vi "Begin.vi"() -> (0 "error out":errorcluster)   [LabVIEW 2014]
doc: "Called before other user functions, this VI is expected to open initial I/O refnums, load in file data, and do all program initialization. Notice that the <B>error out</B> terminal is simply used for data flow. Wiring it to other structures or subVIs ensures that this VI runs first."
uses:
  <vilib>/Rock Robotics/WPI/DriverStation/WPI_DriverStationRobotMode2.ctl
  <vilib>/Rock Robotics/WPI/Joystick/WPI_JoystickDeviceEnum.ctl
  <vilib>/Rock Robotics/SystemInterfaces/DIO/FPGA_DIOPWMChannel.ctl
  <vilib>/Rock Robotics/SystemInterfaces/DIO/FPGA_DIOChannel.ctl
  <vilib>/Rock Robotics/WPI/Solenoid/WPI_SolenoidChannel.ctl
  <vilib>/Rock Robotics/SystemInterfaces/AI/FPGA_AIGyroChannel.ctl
  Robot Global Data.vi
  <vilib>/Rock Robotics/Network Tables/SD Write String Array.vi
  <vilib>/Rock Robotics/WPI/MotorControl/WPI_MotorControlOpen Talon.vi
  <vilib>/Rock Robotics/WPI/Counter/WPI_CounterDigitalInputToDigitalSource.vi
  <vilib>/Rock Robotics/WPI/Solenoid/WPI_SolenoidOpenDouble.vi
  Global Variables/Refnum Names.vi
  Global Variables/Calibrations.vi
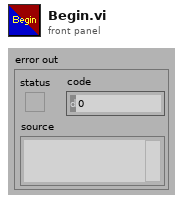
[diagram p1: front panel]
types:
  T1 = typedef "FPGA_DIOChannel.ctl" = enum8{"DIO 0", "DIO 1", "DIO 2", "DIO 3", "DIO 4", "DIO 5", "DIO 6", "DIO 7", "DIO 8", "DIO 9", "DIO MXP 0", "DIO MXP 1", "DIO MXP 2", "DIO MXP 3", "DIO MXP 4", "DIO MXP 5", "DIO MXP 6", "DIO MXP 7", "DIO MXP 8", "DIO MXP 9", "DIO MXP 10", "DIO MXP 11", "DIO MXP 12", "DIO MXP 13", "DIO MXP 14", "DIO MXP 15", "Invalid"}
  T2 = typedef "FPGA_DIOPWMChannel.ctl" = enum8{"PWM 0", "PWM 1", "PWM 2", "PWM 3", "PWM 4", "PWM 5", "PWM 6", "PWM 7", "PWM 8", "PWM 9", "PWM MXP 0", "PWM MXP 1", "PWM MXP 2", "PWM MXP 3", "PWM MXP 4", "PWM MXP 5", "PWM MXP 6", "PWM MXP 7", "PWM MXP 8", "PWM MXP 9", "Invalid"}
  T3 = typedef "WPI_JoystickDeviceEnum.ctl" = enum16{"USB 0", "USB 1", "USB 2", "USB 3", "USB 4", "USB 5"}
  T4 = typedef "FPGA_AIGyroChannel.ctl" = enum8{"AI 0", "AI 1", "Invalid"}
  T5 = typedef "WPI_SolenoidChannel.ctl" = enum8{"Solenoid 0", "Solenoid 1", "Solenoid 2", "Solenoid 3", "Solenoid 4", "Solenoid 5", "Solenoid 6", "Solenoid 7", "Invalid"}
  T6 = typedef "WPI_DriverStationRobotMode2.ctl" = enum16{"Autonomous Disabled", "Autonomous Enabled", "Teleop Disabled", "Teleop Enabled", "Disconnected", "Finish", "Test Disabled", "Test Enabled", "Emergency Stopped"}
  T7 = typedef "WPI_MotorControlDeviceRef.ctl" = cluster{"DeviceStatus":errorcluster, "Type":T8, "PWM":cluster{"Controller":T9, "PWM Channel":T2, "DeadBand":T10}, "CAN":cluster{"Device Number":u8, "Control Mode":T11, "Semaphore":T12, "Max Vout":dbl, "TalonSRX Control Mode":T13}, "Invert":bool, "TransformRef":T14, "InvTransformRef":T14}
  T8 = typedef "WPI_MotorControlType.ctl" = enum16{"PWM", "CAN", "CANTalonSRX"}
  T9 = typedef "FPGA_TypedefDigitalModule.ctl" = enum16{"Controller 1"}
  T10 = typedef "WPI_PWMDeadband.ctl" = cluster{"Name":string, "maxPositivePwm":i32, "minPositivePwm":i32, "centerPwm":i32, "maxNegativePwm":i32, "minNegativePwm":i32, "angularRange":u16}
  T11 = typedef "WPI_CANJaguar_ControlMode.ctl" = enum8{"Percent VBus", "Current", "Speed", "Position", "Voltage"}
  T12 = typedef "Semaphore RefNum" = refnum<k1>
  T13 = typedef "WPI_CANTalonSRX_APIControlMode.ctl" = enum8{"Percent VBus", "Speed", "Position", "Slave", "Unchanged / Invalid"}
  T14 = typedef "WPI_PWMTransform_ConPane.ctl" = refnum<vi>
  T15 = typedef "WPI_ServoDeviceRef.ctl" = cluster{"DeviceStatus":errorcluster, "Controller":T9, "PWM Channel":T2, "DeadBand":T10}
  T16 = typedef "WPI_JoystickDevRef.ctl" = cluster{"Device":T3}
  T17 = typedef "WPI_DigitalInputDevRef.ctl" = cluster{"DevStatus":errorcluster, "DIO Channel":T1, "Controller":T9}
  T18 = typedef "FPGA_CounterEncoderSourceConvertionLVSourceType.ctl" = cluster{"DevStatus":errorcluster, "AnalogTriggerMode?":bool, "DigitalMode":cluster{"Controller":T9, "DIO Channel":T19}, "AnalogTriggerMode":cluster{"AnalogTriggerIndex":T20, "OutputType":T21}}
  T19 = typedef "FPGA_DIODigitalSourceChannel.ctl" = enum8{"DIO 0", "DIO 1", "DIO 2", "DIO 3", "DIO 4", "DIO 5", "DIO 6", "DIO 7", "DIO 8", "DIO 9", "DIO MXP 0", "DIO MXP 1", "DIO MXP 2", "DIO MXP 3", "DIO MXP 4", "DIO MXP 5", "DIO MXP 6", "DIO MXP 7", "DIO MXP 8", "DIO MXP 9", "DIO MXP 10", "DIO MXP 11", "DIO MXP 12", "DIO MXP 13", "DIO MXP 14", "DIO MXP 15", "Disabled"}
  T20 = typedef "FPGA_AnalogTriggerIndex.ctl" = enum8{"Trig 0", "Trig 1", "Trig 2", "Trig 3", "Trig 4", "Trig 5", "Trig 6", "Trig 7", "Invalid"}
  T21 = typedef "FPGA_AnalogTriggerOutType.ctl" = enum16{"InWindow", "TriggerState", "Rising", "Falling"}
  T22 = typedef "WPI_EncoderDevRef.ctl" = cluster{"DevStatus":errorcluster, "EncoderIndex":T23, "CounterIndex":T24, "DistancePerCount":dbl, "Decoding Type":T25}
  T23 = typedef "FPGA_EncoderIdx.ctl" = enum8{"Enc 0", "Enc 1", "Enc 2", "Enc 3", "Enc 4", "Enc 5", "Enc 6", "Enc 7", "Invalid"}
  T24 = typedef "FPGA_CounterCtrSystemIndex.ctl" = enum8{"Ctr 0", "Ctr 1", "Ctr 2", "Ctr 3", "Ctr 4", "Ctr 5", "Ctr 6", "Ctr 7", "Invalid"}
  T25 = typedef "WPI_EncoderType.ctl" = enum16{"1x", "2x", "4x"}
  T26 = typedef "WPI_SolenoidDevRef.ctl" = cluster{"DevStatus":errorcluster, "Pneumatics Control Module":u8, "Forward Solenoid Channel":T5, "Reverse Solenoid Channel":T5}
  T27 = typedef "WPI_GyroDevRef.ctl" = cluster{"DevStatus":errorcluster, "Analog Module":T28, "Analog Channel":T29, "Offset":dbl, "Gain (VoltsPerDegree/Second)":dbl}
  T28 = typedef "FPGA_TypedefAnalogModule.ctl" = enum16{"Controller 1"}
  T29 = typedef "FPGA_AIChannel.ctl" = enum8{"AI 0", "AI 1", "AI 2", "AI 3", "AI MXP 0", "AI MXP 1", "AI MXP 2", "AI MXP 3", "Invalid"}
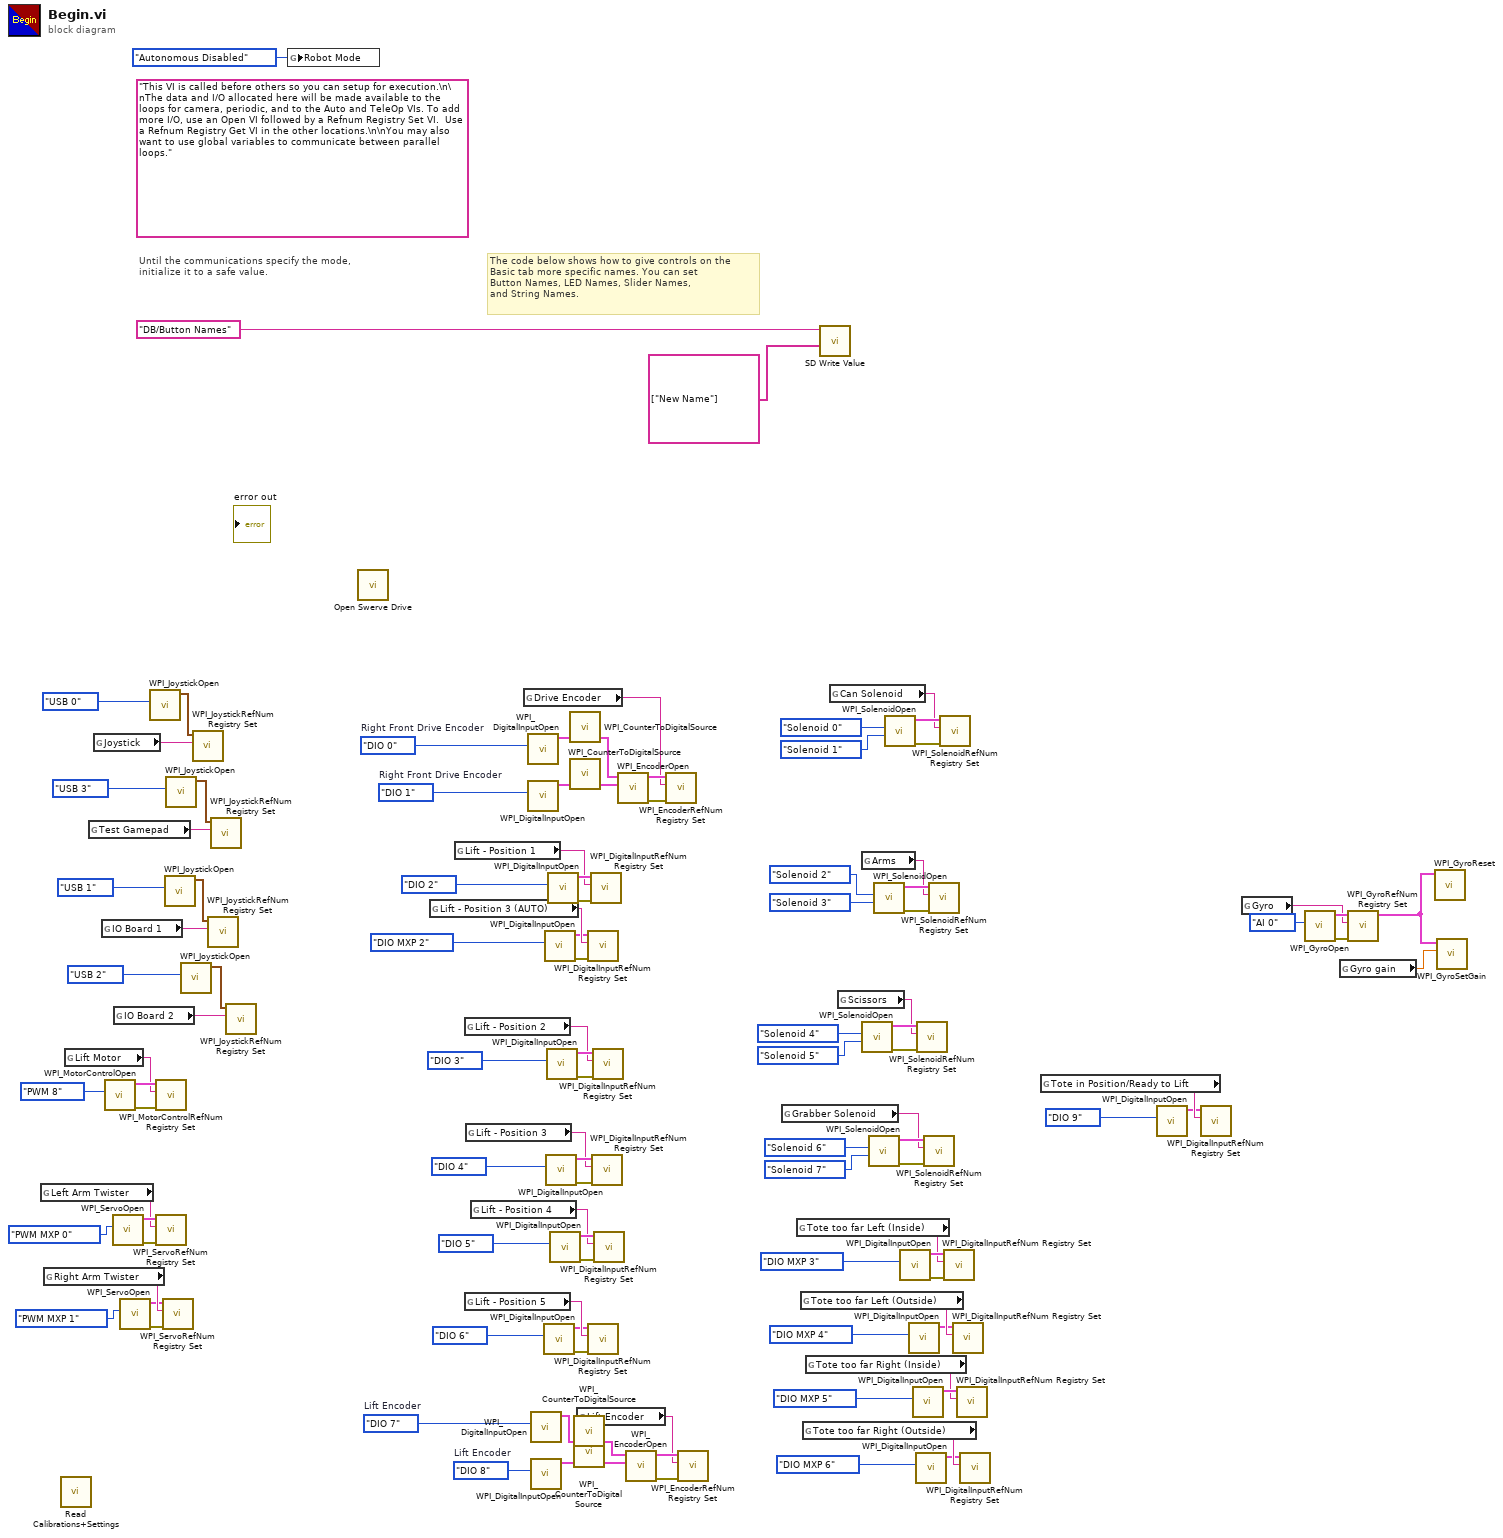
[diagram p0: block diagram]
diagram:
  w75 = FPGA_DIOChannel."DIO 8"  # Lift Encoder
  w74 = FPGA_DIOChannel."DIO 7"  # Lift Encoder
  w96 = FPGA_DIOChannel."DIO 1"  # Right Front Drive Encoder
  w95 = FPGA_DIOChannel."DIO 0"  # Right Front Drive Encoder
  (unwired) "This VI is called before others so you can setup for execution.\n\nThe data and I/O allocated here will be made available to the loops for camera, periodic, and to the Auto and TeleOp VIs. To add more I/O, use an Open VI followed by a Refnum Registry Set VI.  Use a Refnum Registry Get VI in the other locations.\n\nYou may also want to use global variables to communicate between parallel loops."
  # "The code below shows how to give controls on the\nBasic tab more specific names. You can set\nButton Names, LED Names, Slider Names,\nand String Names."
  # "Until the communications specify the mode,\ninitialize it to a safe value."
  n1 = global read "Refnum Names.vi" "Left Arm Twister"() -> (w98:string)
  n2 = global read "Refnum Names.vi" "Right Arm Twister"() -> (w18:string)
  n3 = call "Read Calibrations+Settings.vi"() -> ()  [unwired: 12 in]
  n4 = global read "Refnum Names.vi" "Lift Motor"() -> (w97:string)
  n5 = global read "Refnum Names.vi" "Test Gamepad"() -> (w105:string)
  n6 = global read "Refnum Names.vi" "Joystick"() -> (w103:string)
  n7 = global read "Refnum Names.vi" "IO Board 1"() -> (w26:string)
  n8 = call-poly <vilib>:"WPI_MotorControlOpen.vi"("PWM Channel"=FPGA_DIOPWMChannel."PWM 8") -> ("error out"=w100:errorcluster, "MotorControlDeviceRef"=w101:T7)  [unwired: 9 in]
  n9 = call <vilib>:"WPI_ServoOpen.vi"("PWM Channel"=FPGA_DIOPWMChannel."PWM MXP 0") -> ("error out"=w42:errorcluster, "ServoDeviceRef"=w99:T15)  [unwired: 9 in]
  n10 = global read "Refnum Names.vi" "IO Board 2"() -> (w24:string)
  n11 = call <vilib>:"WPI_ServoOpen.vi"("PWM Channel"=FPGA_DIOPWMChannel."PWM MXP 1") -> ("error out"=w20:errorcluster, "ServoDeviceRef"=w17:T15)  [unwired: 9 in]
  n12 = call <vilib>:"WPI_JoystickOpen.vi"("JoystickDevice"=WPI_JoystickDeviceEnum."USB 0") -> ("JoystickDevRef"=w104:T16)  [unwired: 10 in]
  n13 = call <vilib>:"WPI_MotorControlRefNum Registry Set.vi"("error in (no error)"=w100, "refnum name"=w97, "MotorControlDevRef"=w101) -> ()  [unwired: 7 in, 2 out]
  n14 = call <vilib>:"WPI_ServoRefNum Registry Set.vi"("error in (no error)"=w42, "refnum name"=w98, "ServoDeviceRef"=w99) -> ()  [unwired: 7 in, 2 out]
  n15 = call <vilib>:"WPI_ServoRefNum Registry Set.vi"("error in (no error)"=w20, "refnum name"=w18, "ServoDeviceRef"=w17) -> ()  [unwired: 7 in, 2 out]
  n16 = call <vilib>:"WPI_JoystickOpen.vi"("JoystickDevice"=WPI_JoystickDeviceEnum."USB 1") -> ("JoystickDevRef"=w25:T16)  [unwired: 10 in]
  n17 = call <vilib>:"WPI_JoystickOpen.vi"("JoystickDevice"=WPI_JoystickDeviceEnum."USB 3") -> ("JoystickDevRef"=w106:T16)  [unwired: 10 in]
  n18 = call <vilib>:"WPI_JoystickOpen.vi"("JoystickDevice"=WPI_JoystickDeviceEnum."USB 2") -> ("JoystickDevRef"=w23:T16)  [unwired: 10 in]
  n19 = call <vilib>:"WPI_JoystickRefNum Registry Set.vi"("refnum name"=w103, "JoystickDevRef"=w104) -> ()  [unwired: 8 in, 2 out]
  n20 = call <vilib>:"WPI_JoystickRefNum Registry Set.vi"("refnum name"=w26, "JoystickDevRef"=w25) -> ()  [unwired: 8 in, 2 out]
  n21 = call <vilib>:"WPI_JoystickRefNum Registry Set.vi"("refnum name"=w105, "JoystickDevRef"=w106) -> ()  [unwired: 8 in, 2 out]
  n22 = call <vilib>:"WPI_JoystickRefNum Registry Set.vi"("refnum name"=w24, "JoystickDevRef"=w23) -> ()  [unwired: 8 in, 2 out]
  n23 = global write "Robot Global Data.vi" "Robot Mode"(WPI_DriverStationRobotMode2."Autonomous Disabled" ("Robot Mode")) -> ()
  n24 = call "Open Swerve Drive.vi"() -> ()  [unwired: 12 in]
  n25 = global read "Refnum Names.vi" "Lift - Position 3 (AUTO)"() -> (w16:string)
  n26 = global read "Refnum Names.vi" "Lift - Position 1"() -> (w41:string)
  n27 = global read "Refnum Names.vi" "Lift - Position 2"() -> (w40:string)
  n28 = global read "Refnum Names.vi" "Lift - Position 5"() -> (w37:string)
  n29 = global read "Refnum Names.vi" "Lift - Position 3"() -> (w39:string)
  n30 = global read "Refnum Names.vi" "Lift - Position 4"() -> (w38:string)
  n31 = global read "Refnum Names.vi" "Drive Encoder"() -> (w88:string)
  n32 = call <vilib>:"WPI_DigitalInputOpen.vi"("DIO Channel"=w95) -> ("DigitalInputDevRef"=w93:T17)  [unwired: 2 in, 8 out]
  n33 = call <vilib>:"WPI_DigitalInputOpen.vi"("DIO Channel"=w96) -> ("DigitalInputDevRef"=w94:T17)  [unwired: 2 in, 8 out]
  n34 = call <vilib>:"WPI_DigitalInputOpen.vi"("DIO Channel"=w74) -> ("DigitalInputDevRef"=w72:T17)  [unwired: 2 in, 8 out]
  n35 = call <vilib>:"WPI_DigitalInputOpen.vi"("DIO Channel"=w75) -> ("DigitalInputDevRef"=w73:T17)  [unwired: 2 in, 8 out]
  n36 = call <vilib>:"WPI_DigitalInputOpen.vi"("DIO Channel"=FPGA_DIOChannel."DIO 6") -> ("error out"=w35:errorcluster, "DigitalInputDevRef"=w34:T17)  [unwired: 9 in]
  n37 = call <vilib>:"WPI_DigitalInputOpen.vi"("DIO Channel"=FPGA_DIOChannel."DIO MXP 2") -> ("error out"=w14:errorcluster, "DigitalInputDevRef"=w13:T17)  [unwired: 9 in]
  n38 = call <vilib>:"WPI_DigitalInputOpen.vi"("DIO Channel"=FPGA_DIOChannel."DIO 4") -> ("error out"=w80:errorcluster, "DigitalInputDevRef"=w81:T17)  [unwired: 9 in]
  n39 = call <vilib>:"WPI_DigitalInputOpen.vi"("DIO Channel"=FPGA_DIOChannel."DIO 3") -> ("error out"=w83:errorcluster, "DigitalInputDevRef"=w84:T17)  [unwired: 9 in]
  n40 = call <vilib>:"WPI_DigitalInputOpen.vi"("DIO Channel"=FPGA_DIOChannel."DIO 2") -> ("error out"=w86:errorcluster, "DigitalInputDevRef"=w87:T17)  [unwired: 9 in]
  n41 = call <vilib>:"WPI_DigitalInputOpen.vi"("DIO Channel"=FPGA_DIOChannel."DIO 5") -> ("error out"=w77:errorcluster, "DigitalInputDevRef"=w78:T17)  [unwired: 9 in]
  n42 = call-poly <vilib>:"WPI_CounterToDigitalSource.vi"("DigitalInputDevRef"=w93) -> ("Digital Source"=w92:T18)  [unwired: 6 out]
  n43 = call-poly <vilib>:"WPI_CounterToDigitalSource.vi"("DigitalInputDevRef"=w94) -> ("Digital Source"=w91:T18)  [unwired: 6 out]
  n44 = call-poly <vilib>:"WPI_CounterToDigitalSource.vi"("DigitalInputDevRef"=w72) -> ("Digital Source"=w71:T18)  [unwired: 6 out]
  n45 = call-poly <vilib>:"WPI_CounterToDigitalSource.vi"("DigitalInputDevRef"=w73) -> ("Digital Source"=w70:T18)  [unwired: 6 out]
  n46 = global read "Refnum Names.vi" "Lift Encoder"() -> (w67:string)
  n47 = call <vilib>:"WPI_DigitalInputRefNum Registry Set.vi"("error in (no error)"=w14, "refnum name"=w16, "DigitalInputDevRef"=w13) -> ()  [unwired: 7 in, 2 out]
  n48 = call <vilib>:"WPI_DigitalInputRefNum Registry Set.vi"("error in (no error)"=w35, "refnum name"=w37, "DigitalInputDevRef"=w34) -> ()  [unwired: 7 in, 2 out]
  n49 = call <vilib>:"WPI_DigitalInputRefNum Registry Set.vi"("error in (no error)"=w86, "refnum name"=w41, "DigitalInputDevRef"=w87) -> ()  [unwired: 7 in, 2 out]
  n50 = call <vilib>:"WPI_DigitalInputRefNum Registry Set.vi"("error in (no error)"=w80, "refnum name"=w39, "DigitalInputDevRef"=w81) -> ()  [unwired: 7 in, 2 out]
  n51 = call <vilib>:"WPI_DigitalInputRefNum Registry Set.vi"("error in (no error)"=w83, "refnum name"=w40, "DigitalInputDevRef"=w84) -> ()  [unwired: 7 in, 2 out]
  n52 = call <vilib>:"WPI_DigitalInputRefNum Registry Set.vi"("error in (no error)"=w77, "refnum name"=w38, "DigitalInputDevRef"=w78) -> ()  [unwired: 7 in, 2 out]
  n53 = call <vilib>:"WPI_EncoderOpen.vi"("BSource"=w91, "ASource"=w92) -> ("error out"=w89:errorcluster, "EncoderDevRef"=w90:T22)  [unwired: 6 in, 2 out]
  n54 = call <vilib>:"WPI_EncoderOpen.vi"("BSource"=w70, "ASource"=w71) -> ("error out"=w68:errorcluster, "EncoderDevRef"=w69:T22)  [unwired: 6 in, 2 out]
  n55 = call <vilib>:"WPI_EncoderRefNum Registry Set.vi"("error in (no error)"=w89, "refnum name"=w88, "EncoderDevRef"=w90) -> ()  [unwired: 7 in, 2 out]
  n56 = call <vilib>:"WPI_EncoderRefNum Registry Set.vi"("error in (no error)"=w68, "refnum name"=w67, "EncoderDevRef"=w69) -> ()  [unwired: 7 in, 2 out]
  n57 = global read "Refnum Names.vi" "Grabber Solenoid"() -> (w44:string)
  n58 = global read "Refnum Names.vi" "Tote too far Left (Inside)"() -> (w30:string)
  n59 = global read "Refnum Names.vi" "Tote too far Left (Outside)"() -> (w12:string)
  n60 = global read "Refnum Names.vi" "Tote too far Right (Outside)"() -> (w6:string)
  n61 = global read "Refnum Names.vi" "Tote too far Right (Inside)"() -> (w7:string)
  n62 = call-poly <vilib>:"SD Write Value.vi"("String Array"=string[] ["New Name"], "Name"="DB/Button Names") -> ()  [unwired: 8 in, 2 out]
  n63 = global read "Refnum Names.vi" "Can Solenoid"() -> (w59:string)
  n64 = global read "Refnum Names.vi" "Scissors"() -> (w49:string)
  n65 = global read "Refnum Names.vi" "Arms"() -> (w54:string)
  n66 = call-poly <vilib>:"WPI_SolenoidOpen.vi"("Reverse Solenoid Channel"=WPI_SolenoidChannel."Solenoid 5", "Forward Solenoid Channel"=WPI_SolenoidChannel."Solenoid 4" ("Solenoid Channel")) -> ("error out"=w53:errorcluster, "SolenoidDevRef"=w52:T26)  [unwired: 8 in]
  n67 = call-poly <vilib>:"WPI_SolenoidOpen.vi"("Reverse Solenoid Channel"=WPI_SolenoidChannel."Solenoid 7", "Forward Solenoid Channel"=WPI_SolenoidChannel."Solenoid 6" ("Solenoid Channel")) -> ("error out"=w48:errorcluster, "SolenoidDevRef"=w47:T26)  [unwired: 8 in]
  n68 = call-poly <vilib>:"WPI_SolenoidOpen.vi"("Reverse Solenoid Channel"=WPI_SolenoidChannel."Solenoid 3", "Forward Solenoid Channel"=WPI_SolenoidChannel."Solenoid 2" ("Solenoid Channel")) -> ("error out"=w58:errorcluster, "SolenoidDevRef"=w57:T26)  [unwired: 8 in]
  n69 = call-poly <vilib>:"WPI_SolenoidOpen.vi"("Reverse Solenoid Channel"=WPI_SolenoidChannel."Solenoid 1", "Forward Solenoid Channel"=WPI_SolenoidChannel."Solenoid 0" ("Solenoid Channel")) -> ("error out"=w63:errorcluster, "SolenoidDevRef"=w62:T26)  [unwired: 8 in]
  n70 = call <vilib>:"WPI_DigitalInputOpen.vi"("DIO Channel"=FPGA_DIOChannel."DIO MXP 3") -> ("error out"=w32:errorcluster, "DigitalInputDevRef"=w33:T17)  [unwired: 9 in]
  n71 = call <vilib>:"WPI_DigitalInputOpen.vi"("DIO Channel"=FPGA_DIOChannel."DIO MXP 4") -> ("DigitalInputDevRef"=w10:T17)  [unwired: 9 in, 1 out]
  n72 = call <vilib>:"WPI_DigitalInputOpen.vi"("DIO Channel"=FPGA_DIOChannel."DIO MXP 5") -> ("DigitalInputDevRef"=w9:T17)  [unwired: 9 in, 1 out]
  n73 = call <vilib>:"WPI_DigitalInputOpen.vi"("DIO Channel"=FPGA_DIOChannel."DIO MXP 6") -> ("DigitalInputDevRef"=w4:T17)  [unwired: 9 in, 1 out]
  n74 = call <vilib>:"WPI_SolenoidRefNum Registry Set.vi"("error in (no error)"=w53, "refnum name"=w49, "SolenoidDevRef"=w52) -> ()  [unwired: 7 in, 2 out]
  n75 = call <vilib>:"WPI_SolenoidRefNum Registry Set.vi"("error in (no error)"=w48, "refnum name"=w44, "SolenoidDevRef"=w47) -> ()  [unwired: 7 in, 2 out]
  n76 = call <vilib>:"WPI_SolenoidRefNum Registry Set.vi"("error in (no error)"=w58, "refnum name"=w54, "SolenoidDevRef"=w57) -> ()  [unwired: 7 in, 2 out]
  n77 = call <vilib>:"WPI_SolenoidRefNum Registry Set.vi"("error in (no error)"=w63, "refnum name"=w59, "SolenoidDevRef"=w62) -> ()  [unwired: 7 in, 2 out]
  n78 = call <vilib>:"WPI_DigitalInputRefNum Registry Set.vi"("error in (no error)"=w32, "refnum name"=w30, "DigitalInputDevRef"=w33) -> ()  [unwired: 7 in, 2 out]
  n79 = call <vilib>:"WPI_DigitalInputRefNum Registry Set.vi"("refnum name"=w12, "DigitalInputDevRef"=w10) -> ()  [unwired: 8 in, 2 out]
  n80 = call <vilib>:"WPI_DigitalInputRefNum Registry Set.vi"("refnum name"=w7, "DigitalInputDevRef"=w9) -> ()  [unwired: 8 in, 2 out]
  n81 = call <vilib>:"WPI_DigitalInputRefNum Registry Set.vi"("refnum name"=w6, "DigitalInputDevRef"=w4) -> ()  [unwired: 8 in, 2 out]
  n82 = global read "Refnum Names.vi" "Tote in Position/Ready to Lift"() -> (w3:string)
  n83 = call <vilib>:"WPI_DigitalInputOpen.vi"("DIO Channel"=FPGA_DIOChannel."DIO 9") -> ("DigitalInputDevRef"=w1:T17)  [unwired: 9 in, 1 out]
  n84 = call <vilib>:"WPI_DigitalInputRefNum Registry Set.vi"("refnum name"=w3, "DigitalInputDevRef"=w1) -> ()  [unwired: 8 in, 2 out]
  n85 = global read "Refnum Names.vi" "Gyro"() -> (w64:string)
  n86 = call <vilib>:"WPI_GyroOpen.vi"("Analog Channel"=FPGA_AIGyroChannel."AI 0") -> ("error out"=w66:errorcluster, "GyroDevRef"=w65:T27)  [unwired: 8 in, 1 out]
  n87 = global read "Calibrations.vi" "Gyro gain"() -> (w27:dbl)
  n88 = call <vilib>:"WPI_GyroRefNum Registry Set.vi"("error in (no error)"=w66, "refnum name"=w64, "GyroDevRef"=w65) -> ("GyroDevRef"=w28:T27)  [unwired: 7 in, 1 out]
  n89 = call <vilib>:"WPI_GyroReset.vi"("GyroDevRef"=w28) -> ()  [unwired: 9 in, 2 out]
  n90 = call <vilib>:"WPI_GyroSetGain.vi"("Gain (VoltsPerDegree/Second)"=w27, "GyroDevRef"=w28) -> ()  [unwired: 8 in, 2 out]
